vi "Config Crosslinking Test.vi"() -> (0 "error out":errorcluster, 2 "Editor crosslinked?":bool, 3 "Runtime crosslinked?":bool)   [LabVIEW 2013, in "Tagbus PID Module tests.lvlib"]
uses:
  Tagbus PID Module tests.lvlib
panel:
  out "Array 2":path[](array[path])
  out "Array":path[](array[path])
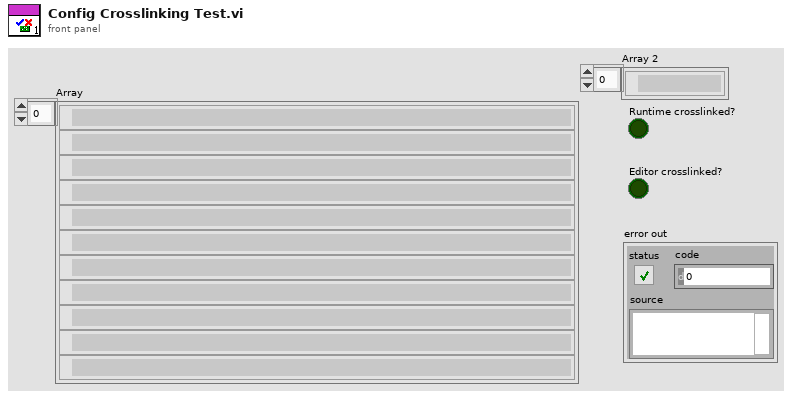
[diagram p1: front panel]
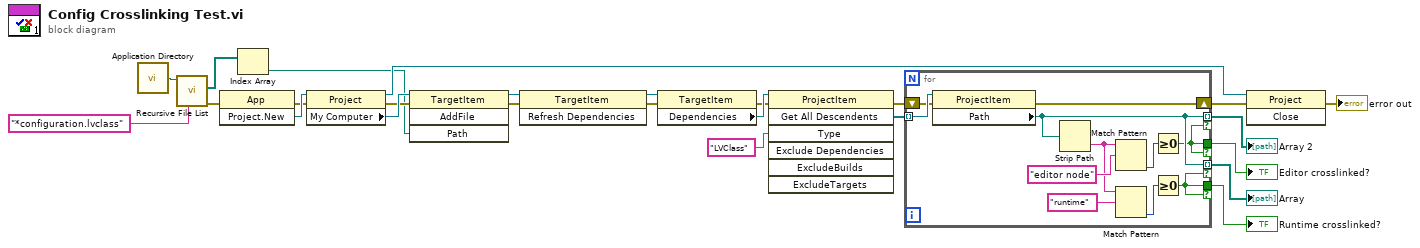
[diagram p0: block diagram]
diagram:
  n1 = call <vilib>:"Application Directory.vi"() -> ("Application Directory"=w8:path)
  n2 = call <vilib>:"Recursive File List.vi"("pattern"="*configuration.lvclass", "Folder Path"=w8) -> ("error out"=w4:errorcluster, "All Files in Dir"=w6:path[])  [unwired: 5 in, 3 out]
  n3 = invoke class="App" method="Project.New"(error in=w4) -> (error out=w19:errorcluster, "Project:New"=w22:refnum<vi>)  [unwired: 2 in, 1 out]
  n4 = Index Array(array=w6) -> (element=w5:path)  [unwired: 1 in]
  n5 = property class="Project"(reference=w22, error in=w19) -> (reference out=w13:refnum<vi>, error out=w20:errorcluster, "My Computer"=w21:refnum<vi>)
  n6 = invoke class="TargetItem" method="AddFile"(reference=w21, error in=w20, "Path"=w5) -> (reference out=w18:refnum<vi>, error out=w16:errorcluster)  [unwired: 1 in, 2 out]
  n7 = invoke class="TargetItem" method="Refresh Dependencies"(reference=w18, error in=w16) -> (reference out=w17:refnum<vi>, error out=w15:errorcluster)  [unwired: 1 in, 1 out]
  n8 = property class="TargetItem"(reference=w17, error in=w15) -> (error out=w11:errorcluster, "Dependencies"=w24:refnum<vi>)  [unwired: 1 out]
  n9 = invoke class="ProjectItem" method="Get All Descendents"(reference=w24, error in=w11, "Type"="LVClass") -> (error out=w12:errorcluster, "All Descendents"=w23:refnum<vi>[])  [unwired: 4 in, 5 out]
  n10 = for {
    tunnel: w23 -> [w36] mode=indexing
    shift-right: [w35] -> w14
    shift-left: w12 -> [w34]
    tunnel: [w27] -> w9 if=w27
    tunnel: [w26] -> w3 if=w26
    tunnel: [w28] -> w2 mode=indexing if=w26
    tunnel: [w28] -> w1 mode=indexing if=w27
    n11 = property class="ProjectItem"(reference=w36, error in=w34) -> (error out=w35:errorcluster, "Path"=w28:path)  [unwired: 1 out]
    n12 = Strip Path(path=w28) -> (name=w31:string)  [unwired: 1 out]
    n13 = Match Pattern(string=w31, regular expression="editor node") -> (offset past match=w32:i32)  [unwired: 1 in, 3 out]
    n14 = Match Pattern(string=w31, regular expression="runtime") -> (offset past match=w29:i32)  [unwired: 1 in, 3 out]
    n15 = Greater Or Equal To 0?(x=w32) -> (x >= 0?=w27:bool)
    n16 = Greater Or Equal To 0?(x=w29) -> (x >= 0?=w26:bool)
  }
  "Editor crosslinked?" <- w9
  "Runtime crosslinked?" <- w3
  "Array" <- w2
  "Array 2" <- w1
  n17 = invoke class="Project" method="Close"(reference=w13, error in=w14) -> (error out=→"error out":errorcluster)  [unwired: 1 in, 2 out]
